vi "Replace Array Element.vi"(5 "New Element":variant, 8 "错误输入":errorcluster, 9 "Indices(>=1D)":u32[](array[numeric]), 10 "Index (1D)":u32, 11 "MultiD Array":variant) -> (0 "错误输出":errorcluster, 2 "VMultiD Array":variant)   [LabVIEW 2012, in "TD Tools.lvlib"]
uses:
  TD Tools.lvlib
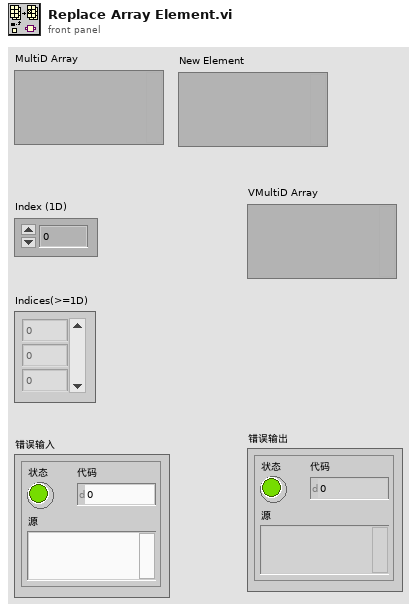
[diagram p1: front panel]
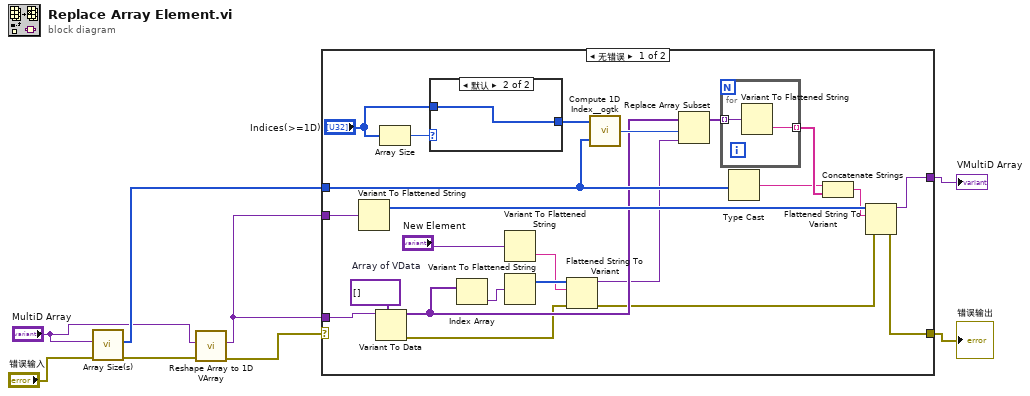
[diagram p0: block diagram]
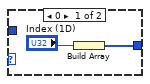
[diagram p2: hidden frame]
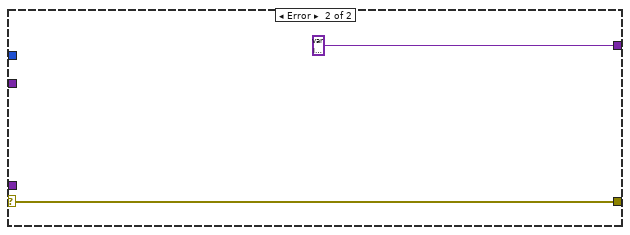
[diagram p3: hidden frame]
diagram:
  n1 = call "Array Size(s).vi"("错误输入"="错误输入", "Array"="MultiD Array") -> ("错误输出"=w6:errorcluster, "Size(s)"=w7:u32[])  [unwired: 7 in, 1 out]
  n2 = call "Reshape Array to 1D VArray.vi"("error in (no error)"=w6, "MultiD Array"="MultiD Array") -> ("error out"=w4:errorcluster, "1D VArray"=w1:variant)  [unwired: 7 in, 1 out]
  n3 = case shown="无错误" w4 {
    selector: w4 -> [_ w38]
    tunnel: [w20 w38] -> w2
    tunnel: w1 -> [w31 _]
    tunnel: w7 -> [w19 _]
    tunnel: [w21 variant ("MultiD Array")] -> w3
    tunnel: w1 -> [w26 _]
    frame No Error {
      w30 = variant[] []  # Array of VData
      n4 = Variant To Flattened String(Variant=w26) -> (1:w23:i16[])  [unwired: 1 out]
      n5 = Variant To Data(type=w30, Variant=w31) -> (data=w17:variant[], error out=w11:errorcluster)  [unwired: 1 in]
      n6 = Array Size(array="Indices(>=1D)") -> (size(s)=w29:i32)
      n7 = case shown="默认" w29 {
        tunnel: [w35 w36] -> w28
        tunnel: "Indices(>=1D)" -> [_ w36]
        frame 0 {
          n8 = Build Array("Index (1D)") -> (w35:u32[])
        }
        frame Default {
        }
      }
      n9 = Index Array(array=w17) -> (element=w16:variant)  [unwired: 1 in]
      n10 = Variant To Flattened String(Variant="New Element") -> (data string=w14:string)  [unwired: 1 out]
      n11 = Variant To Flattened String(Variant=w16) -> (1:w15:i16[])  [unwired: 1 out]
      n12 = Flattened String To Variant(4:w11, 6:w14, 7:w15) -> (0:w12:errorcluster, 3:w13:variant)
      n13 = call <userlib>:"Compute 1D Index__ogtk.vi"("Size(s)"=w19, "Indices"=w28) -> ("1D Index"=w27:i32)
      n14 = Replace Array Subset(array=w17, new element=w13, index=w27) -> (w25:variant[])
      n15 = for {
        tunnel: w25 -> [w33] mode=indexing
        tunnel: [w32] -> w24 mode=indexing
        n16 = Variant To Flattened String(Variant=w33) -> (data string=w32:string)  [unwired: 1 out]
      }
      n17 = Type Cast(x=w19) -> (*(type *) &x=w18:string)  [unwired: 1 in]
      n18 = Concatenate Strings(w18, w24) -> (w22:string)
      n19 = Flattened String To Variant(4:w12, 6:w22, 7:w23) -> (0:w20:errorcluster, 3:w21:variant)
    }
    frame Error {
    }
  }
  "VMultiD Array" <- w3
  "错误输出" <- w2
